vi "ReadTrigger.vi"(8 "error in":errorcluster, 11 "TriggerBox in":refnum<class "TriggerBox.lvclass">) -> (0 "error out":errorcluster, 1 "TriggerArmed":bool, 2 "TriggerFired":bool, 3 "TriggerBox out":refnum<class "TriggerBox.lvclass">)   [LabVIEW 2013, in "TriggerBox.lvclass"]
uses:
  TriggerBox.lvclass
  <vilib>/Utility/error.llb/Error Cluster From Error Code.vi
  <vilib>/rvi/errors/niLvFpgaAdjustHostInterfaceError.vi
  RT/FPGASession/FPGARef.ctl
  <vilib>/rvi/interface/nirviReadWriteControl/nirviReadWriteControl.xnode
  FPGA Bitfiles/HWSWTriggerBox_FPGATarget2_TriggerBox_1zhzIx5zPP8.lvbitx
  FPGAMain.vi
  FPGASessionClass/FPGASession.lvclass
  NiFpgaLv.dll
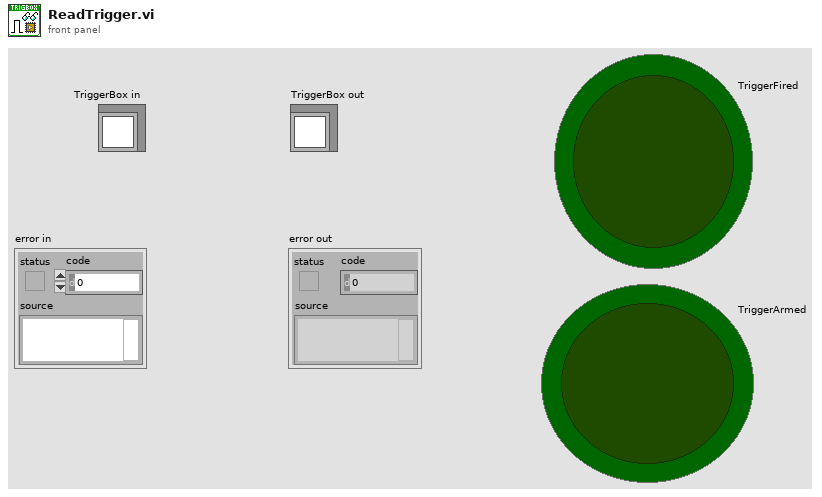
[diagram p1: front panel]
types:
  T1 = typedef "FPGASession.lvclass/FPGARef.ctl" = refnum<k20>
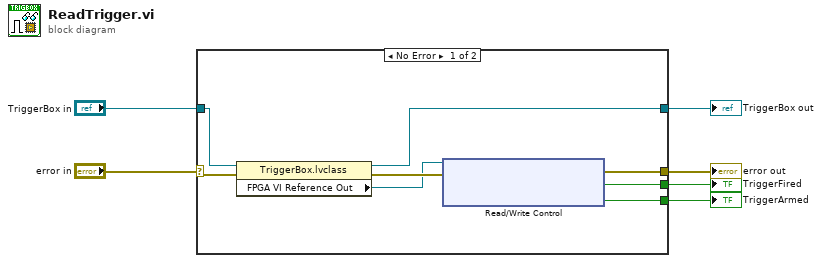
[diagram p0: block diagram]
diagram:
  n1 = case shown="No Error" "error in" {
    selector: "error in" -> [w11 w16]
    tunnel: [w14 w16] -> w3
    tunnel: [w7 w15] -> w4
    tunnel: "TriggerBox in" -> [w10 w15]
    tunnel: [w13 _] -> w2
    tunnel: [w12 _] -> w1
    frame No Error {
      n2 = property class="TriggerBox.lvclass"(reference=w10, error in=w11) -> (reference out=w7:refnum<class "TriggerBox.lvclass">, error out=w9:errorcluster, "FPGA VI Reference Out"=w8:T1)
      n3 = xnode "Read/Write Control"("FPGA VI Reference In"=w8, "error in"=w9) -> ("error out"=w14:errorcluster, "TriggerFired"=w13:bool, "TriggerArmed"=w12:bool)  [unwired: 1 out]
    }
    frame Error {
    }
  }
  "error out" <- w3
  "TriggerBox out" <- w4
  "TriggerFired" <- w2
  "TriggerArmed" <- w1
